vi "HVGEM_AMP_6.2_forDAQ.vi"() -> ()   [LabVIEW 2021]
uses:
  <vilib>/Utility/error.llb/DialogType.ctl
  lib/HVG211.llb/GlobalData.vi
  lib/HVG211.llb/variables.vi
panel:
  in  "path":path=path "Z:/"
  out "refnum":refnum<file>
  out "file open":bool=TRUE caption="Fast"
  in  "ON OLD":bool=TRUE
  out "HV_flag":bool=TRUE
  in  "stop":bool=TRUE caption="Fast"
  out "Currents 2":dbl[](array[numeric]) caption="CURRENTS"
  out "Currents":dbl[](array[numeric]) format="%.2f"
  in  "Trip Control":bool=TRUE caption="SetPreOperational"
  out "OVC":u32[](array[numeric])
  in  "CurrThres":dbl=20.0 caption="uA" min=0.1 max=100.0
  in  "OvflThres":u16=25 caption="number of discharges"
  out "TripCtrl_msg":string="OVCs on 50 samples in 1000 ms:\nTrip if   25 times over   20 uA" caption="INFO_msg"
  in  "dt":u16=20 caption="Time step [ms]" max=5000
  in  "DT":u16=1000 caption="Time window [ms]"
  in  "SpsAcc":bool=TRUE caption="Fast"
  out "Trip Status":u16(ring)=2 items=["DISABLED", "INITIALIZING", "RUNNING", "TRIP"]
  out "slope read":i16=15 caption="Channel" max=2500
  in  "setting 2":i32(ring)=1 items=["TPG", "Planare"]
  out "Currents old":dbl[](array[numeric]) caption="Currents"
  out "Voltages old":dbl[](array[numeric])=[28.0, 28.0, 32.0, 30.0, 29.0, 29.0, 58.0, 0.0, 0.0] caption="Voltages"
  out "sumnew":u16=234
  out "sumold":u16=234
  out "DACOLD":u16[](array[numeric])=[28, 28, 32, 30, 29, 29, 58]
  in  "AVG":u32=100
  out "avg":i16=100 caption="Channel" max=2500
  in  "Slope":u32=15 max=2500
  in  "HV enable switch old":bool=TRUE caption="HV enabled"
  in  "ON":bool
  out "Currents micro":cluster{dbl, dbl, dbl, dbl, dbl, dbl, dbl}(graph)
  out "Wiper":i16[](array[numeric])=[512, 512, 512, 512, 512, 512, 513]
  out "Current_AGC_led":bool
  out "Tramp [s]":u16=5 caption="Channel" max=2500
  out "Tstep [ms]":u16=10 caption="Channel" max=2500
  out "Power Supply Levels":dbl[](array[numeric])=[29.45, 5.357, 3.476, 16.071, 0.384] format="%.1f"
  out "HV enable switch":bool=TRUE caption="HV enabled"
  out "Safety switch":bool=TRUE caption="Cable IN"
  out "FSM_status":u16(ring) items=["IDLE", "RAMPING", "INIT", "ABORTING", "CLEARING", "5", "6", "7", ""]
  out "I_gain_x10":bool[](array[boolean])
  out "HV_on":bool[](array[boolean])=[TRUE, TRUE, TRUE, TRUE, TRUE, TRUE, TRUE, FALSE] caption="HV_ON"
  out "Voltages":dbl[](array[numeric])=[28.0, 28.0, 33.0, 30.0, 29.0, 30.0, 58.0, 0.0, 0.0] caption="VOLTAGES"
  out "TPD_read":bool=TRUE
  out "I_data":cluster{dbl[], dbl[]}[](array[cluster])
  out "V_data":cluster{dbl[], dbl[]}[](array[cluster])
  in  "Ind Gap":dbl=1.0
  in  "Gap 2":dbl=2.0
  in  "Gap 1":dbl=2.0
  in  "Drift Gap":dbl=9.0
  out "STATUS":bool=TRUE
  in  "ID":u8=71
  in  "Limit":u32=2400 min=600 max=3500 step=50
  in  "setting":i32(ring)=4 items=["zero", "test", "field", "600", "900", "1050", "1080", "1090", "1100", "1110", "1120", "1130", "1140", "1160", "1200", "1240", "1260", "1280", "1300", "1320"]
  in  "Apply":bool
  out "time":u32=185445358 format="%#.0f"
  in  "Write data":bool
  out "Run":i32=5
  out "Gain":u32=88
  out "String":string="FILLING  HISTOS"
  out "Vd":dbl=58.0
  out "Vt1":dbl=29.0
  out "Vt2":dbl=33.0
  out "Vi":dbl=28.0
  out "G3":dbl=28.0
  out "G1":dbl=30.0
  out "G2":dbl=30.0
  out "Ed":dbl=0.06444444444444444 format="%.1f"
  out "Ei":dbl=0.28 format="%.1f"
  out "Et2":dbl=0.165 format="%.1f"
  out "Et1":dbl=0.145 format="%.1f"
  out "Fields kV/cm":cluster{dbl, dbl, dbl, dbl}(graph)={0.06444444444444444, 0.145, 0.165, 0.28}
  out "GEM Volt":cluster{dbl, dbl, dbl}(graph)={30.0, 30.0, 28.0}
  out "DACNEW":u16[](array[numeric])=[28, 28, 32, 30, 29, 29, 58]
  out "ERROR":errorcluster={"status"=TRUE, "code"=-10, "source"="Handle is invalid"}
  out "PreOperational":bool
  out "Operational":bool=TRUE
  out "OPERATION ERROR":errorcluster
  out "gi":dbl=100.0 format="%.2f"
  out "gt2":dbl=200.0 format="%.2f"
  out "gt1":dbl=200.0 format="%.2f"
  out "gd":dbl=900.0 format="%.2f"
  in  "Ind":dbl=0.28 caption="Induction Field (kV/cm)" min=0.0 max=10.0 step=0.1 format="%.1f"
  in  "T2":dbl=0.16 caption="Transfer Field 2 (kV/cm)" min=0.0 max=4.0 step=0.1 format="%.1f"
  in  "T1":dbl=0.145 caption="Transfer Field 1(kV/cm)" min=0.0 max=4.0 step=0.1 format="%.1f"
  in  "Drift":dbl=0.06444444444444444 caption="Drift Field (kV/cm)" min=0.0 max=4.0 step=0.1 format="%.2f"
  in  "VG3":i16=28 caption="Vg3 (Volt)" min=0 max=600 step=5
  in  "VG2":i16=30 caption="Vg2 (Volt)" min=0 max=600 step=5
  in  "VG1":i16=29 caption="Vg1 (Volt)" min=0 max=600 step=5
  out "t0":u32=1496531
  # "HV GEM AMP 6.2"
  # "HV ON"
  # "Volt"
  # "kV/cm"
  # "kV/cm"
  # "Volt"
  # "GAP(mm)"
  # "EI         G3       ET2      G2      ET1      G1       ED"
  # "TEMP"
  # "PS1"
  # "PS2"
  # "PS3"
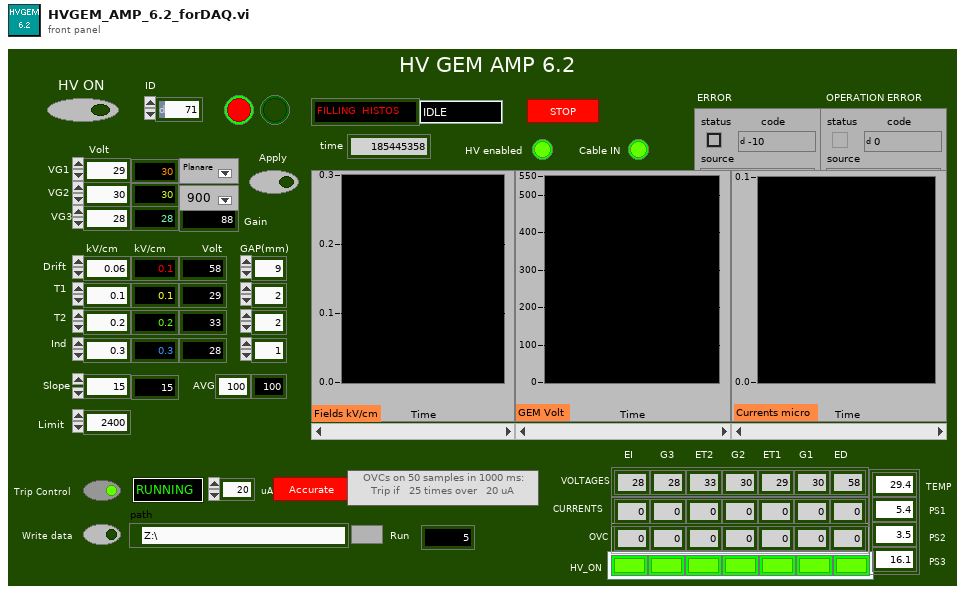
[diagram p1: front panel]
types:
  T1 = enum16{"open", "open or create", "create or replace", "create", "open (read only)"}
  T2 = typedef "DialogType.ctl" = u16
  T3 = cluster{"Safety switch":bool, "HV disable switch":bool, "HV_on":bool[], "I_gain_x10":bool[], "FSM_status":u16, "0x2020":dbl[], "Tstep":u16, "Tramp":u16, "Average":i16, "Current AGC":bool, "Wiper":i16[], "Slope [V/s]":i16}
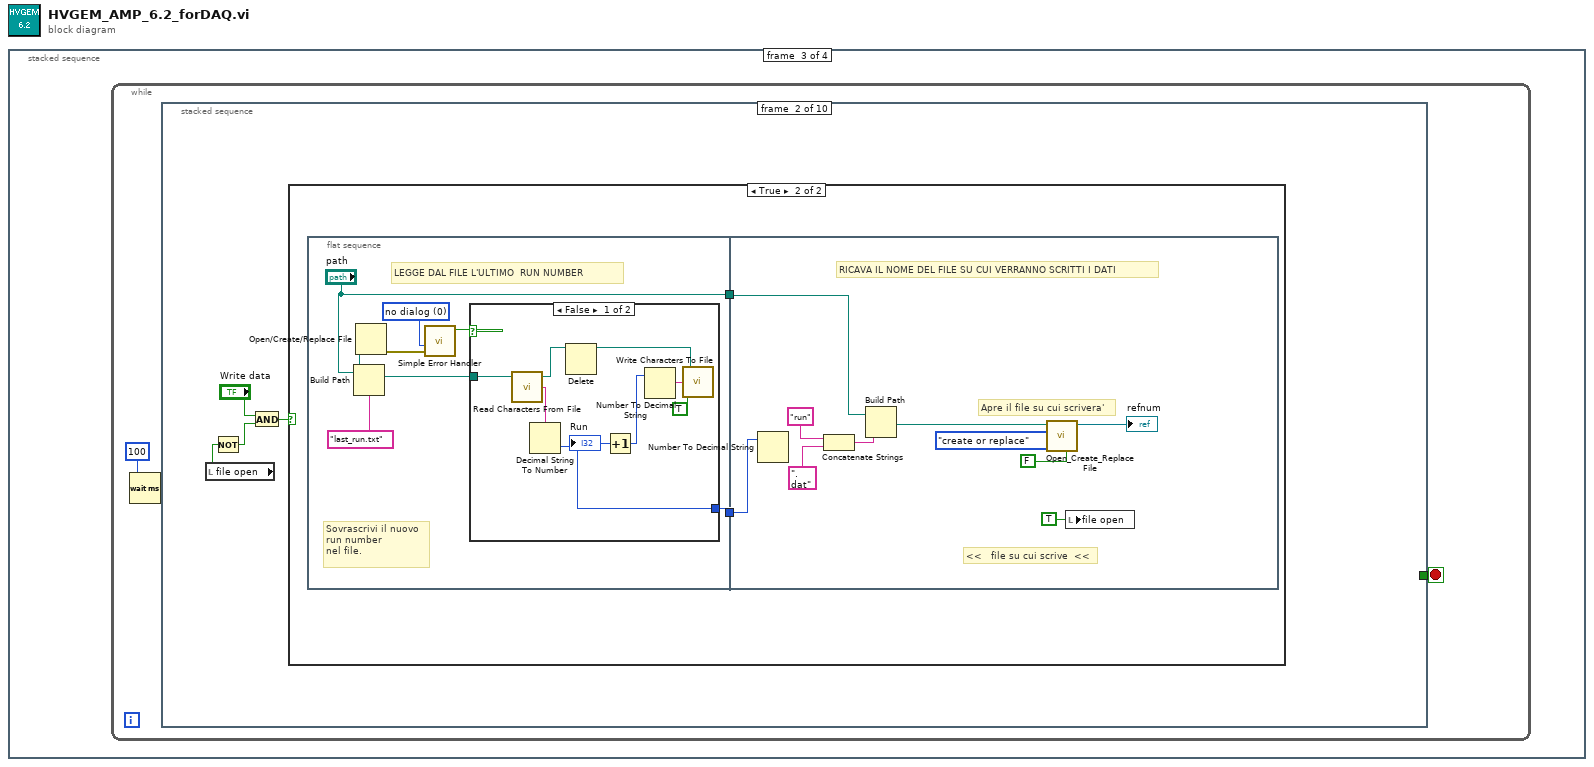
[diagram p0: block diagram]
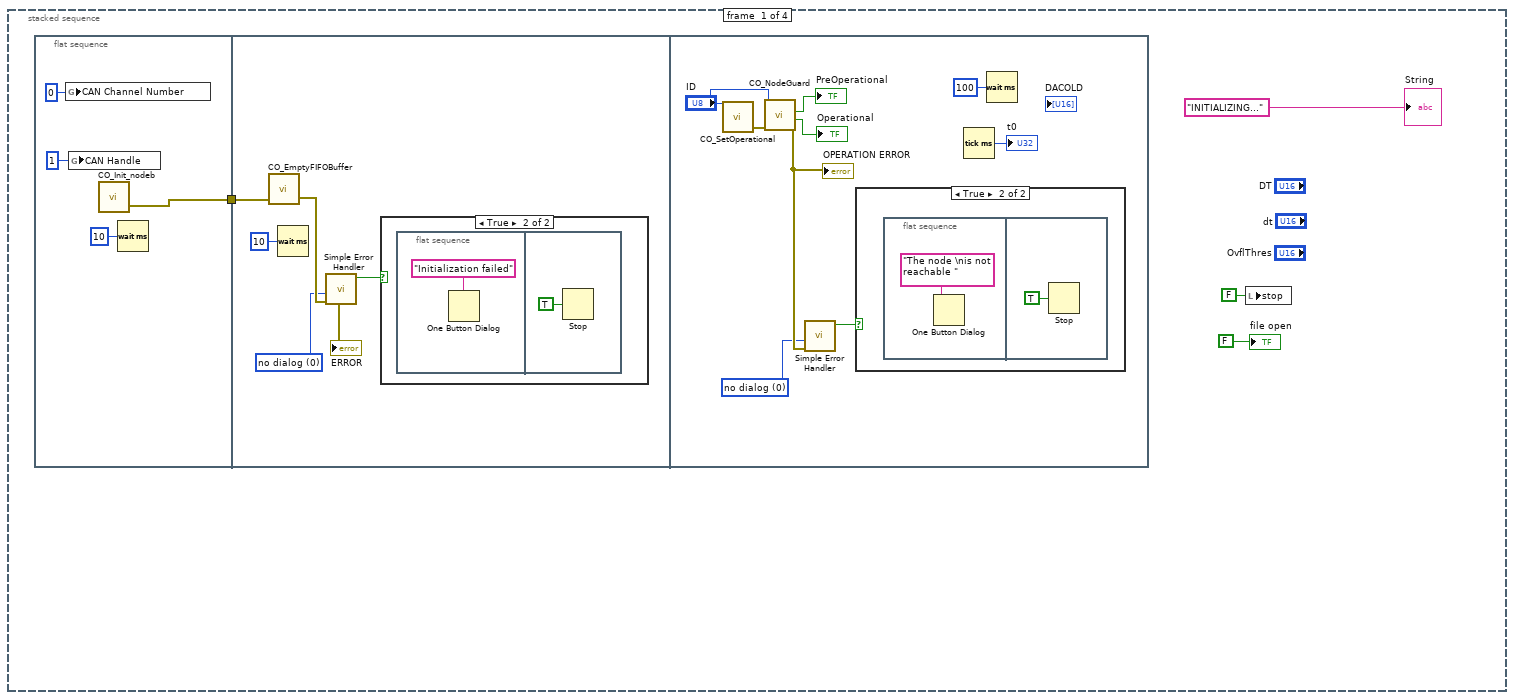
[diagram p2: hidden frame]
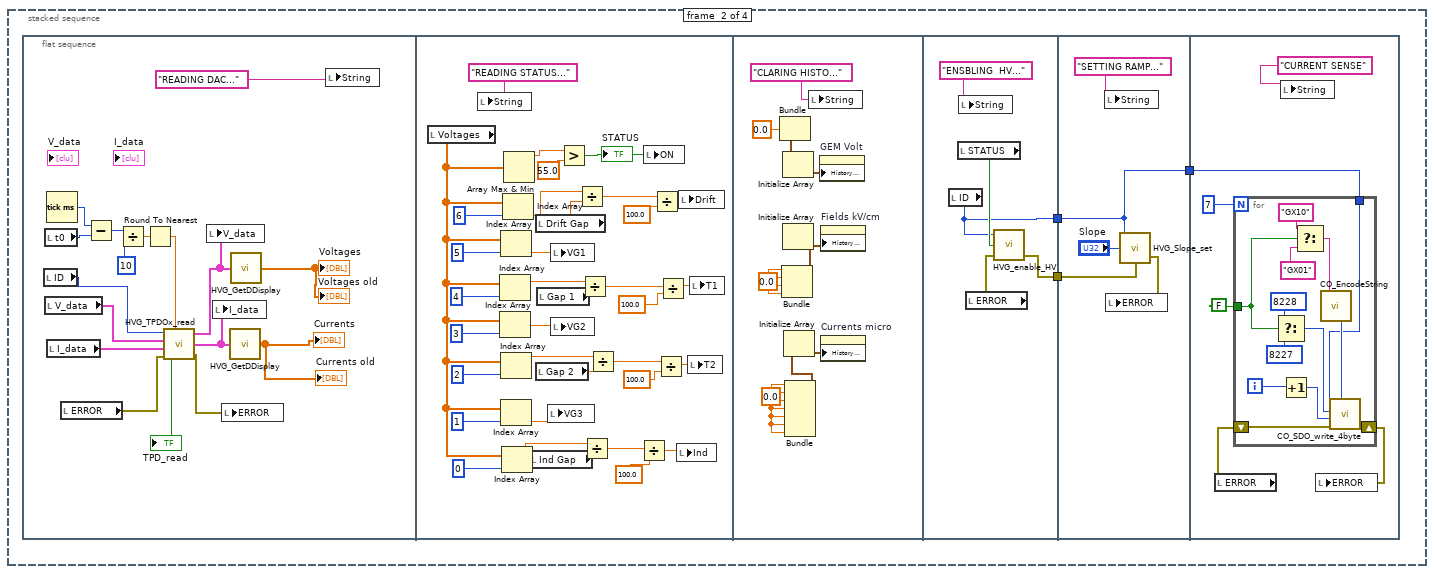
[diagram p5: hidden frame]
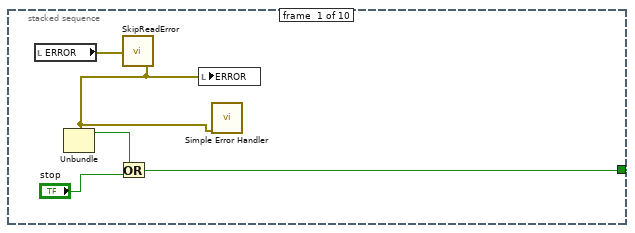
[diagram p6: hidden frame]
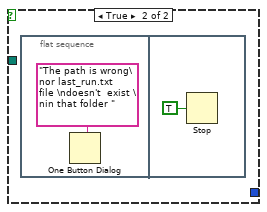
[diagram p8: hidden frame]
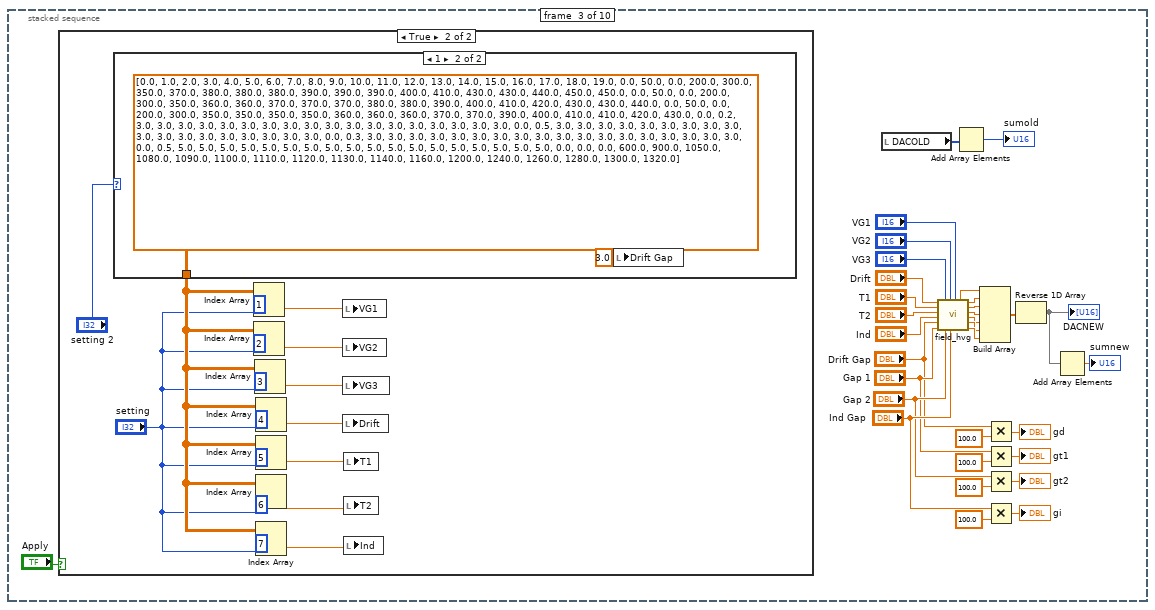
[diagram p9: hidden frame]
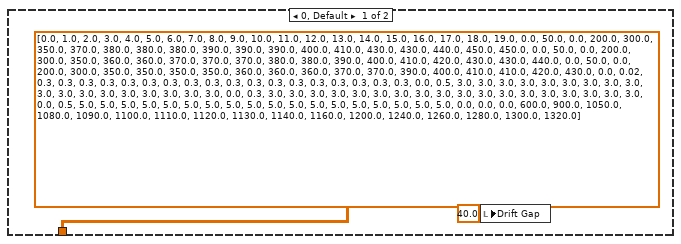
[diagram p11: hidden frame]
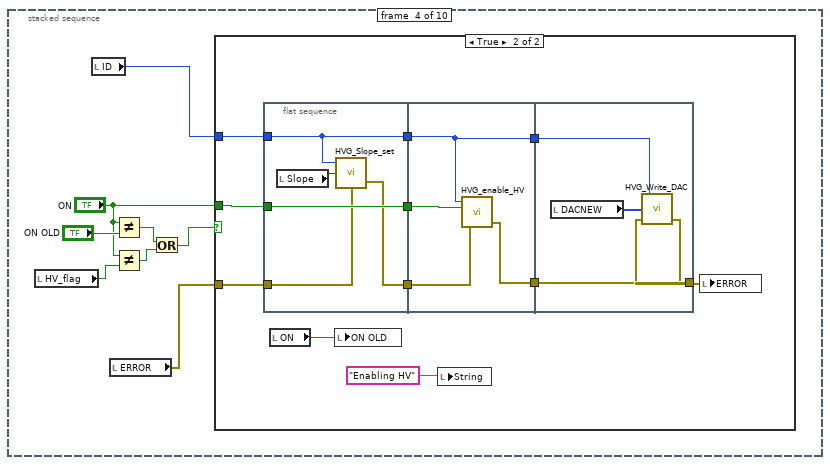
[diagram p12: hidden frame]
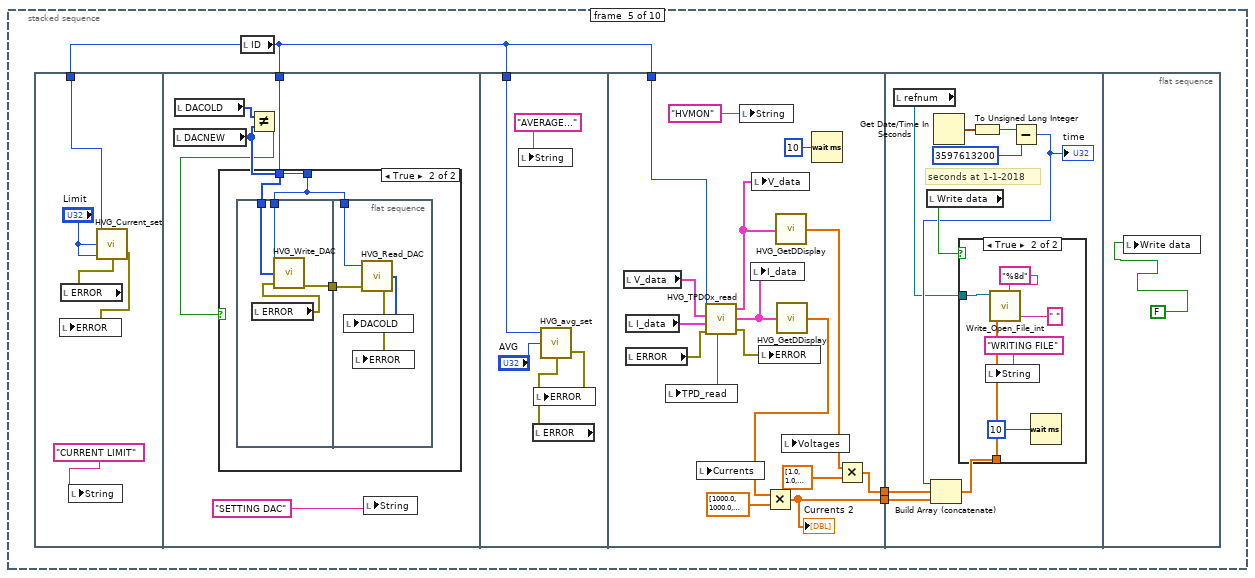
[diagram p14: hidden frame]
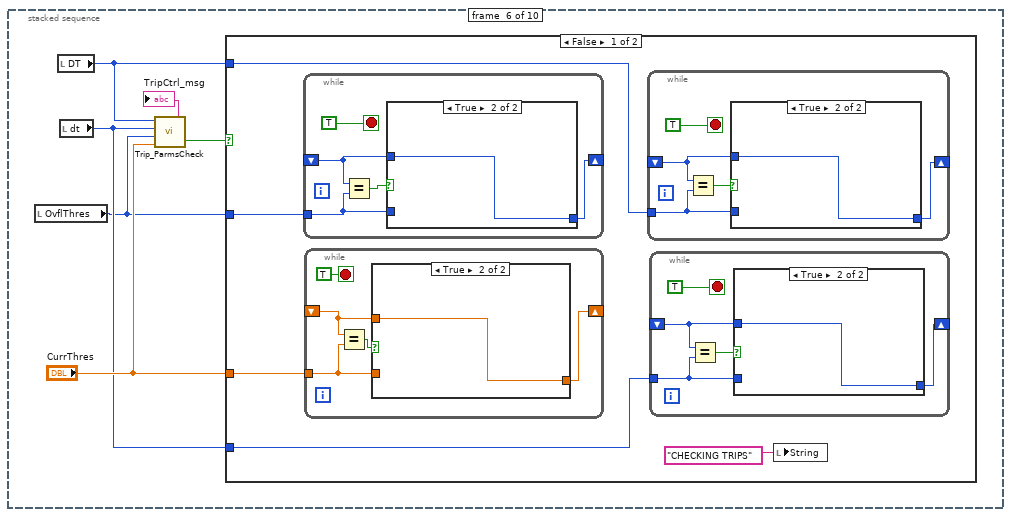
[diagram p17: hidden frame]
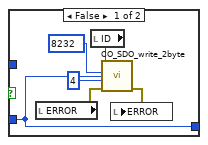
[diagram p18: hidden frame]
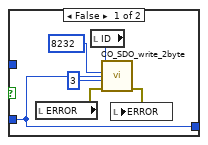
[diagram p19: hidden frame]
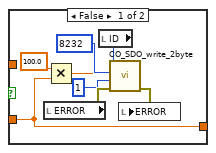
[diagram p20: hidden frame]
diagram:
  n1 = stacked-sequence {
    frame #0 {
      (unwired) FALSE ("Boolean 2")
      n2 = flat-sequence {
        tunnel: [w7] -> w3
        tunnel: w3 -> [w12]
        frame #0 {
          n3 = global write "GlobalData.vi" "CAN Channel Number"(0 ("CAN Handle")) -> ()
          n4 = global write "GlobalData.vi" "CAN Handle"(1 ("CAN Handle")) -> ()
          n5 = call "CO_Init_nodeb.vi"() -> ("error out"=w7:errorcluster)  [unwired: 3 in]
          n6 = Wait (ms)(milliseconds to wait=u32 10) -> ()  [unwired: 1 out]
        }
        frame #1 {
          w9 = T2 0 items=["no dialog", "OK message", "continue or stop message", "OK message + warnings", "continue/stop + warnings"] ("type of dialog (OK msg:1)")
          n7 = call "CO_EmptyFIFOBuffer.vi"("error in"=w12) -> ("error out"=w10:errorcluster)  [unwired: 2 in]
          "ERROR" <- w10
          n8 = Wait (ms)(milliseconds to wait=u32 10) -> ()  [unwired: 1 out]
          n9 = call <vilib>:"Simple Error Handler.vi"("type of dialog (OK msg:1)"=w9, "error in (no error)"=w10) -> ("error?"=w11:bool)  [unwired: 3 in, 4 out]
          n10 = case shown="True" w11 {
            frame False {
            }
            frame True {
              n11 = flat-sequence {
                frame #0 {
                  n12 = One Button Dialog(message="Initialization failed") -> ()  [unwired: 1 in, 1 out]
                }
                frame #1 {
                  n13 = Stop(stop? (T)=TRUE) -> ()
                }
              }
            }
          }
        }
        frame #2 {
          w16 = T2 0 items=["no dialog", "OK message", "continue or stop message", "OK message + warnings", "continue/stop + warnings"] ("type of dialog (OK msg:1)")
          n14 = call "CO_SetOperational.vi"("ID"="ID") -> ("error out"=w21:errorcluster)  [unwired: 4 in]
          n15 = call "CO_NodeGuard.vi"("error in (no error)"=w21, "ID"="ID") -> ("error out"=w18:errorcluster, "Operational"=→"Operational":bool, "PreOperational"=→"PreOperational":bool)  [unwired: 3 in, 2 out]
          "OPERATION ERROR" <- w18
          n16 = call <vilib>:"Simple Error Handler.vi"("type of dialog (OK msg:1)"=w16, "error in (no error)"=w18) -> ("error?"=w17:bool)  [unwired: 3 in, 4 out]
          n17 = case shown="True" w17 {
            frame False {
            }
            frame True {
              n18 = flat-sequence {
                frame #0 {
                  n19 = One Button Dialog(message="The node \nis not reachable ") -> ()  [unwired: 1 in, 1 out]
                }
                frame #1 {
                  n20 = Stop(stop? (T)=TRUE) -> ()
                }
              }
            }
          }
          n21 = Tick Count (ms)() -> (millisecond timer value=→"t0":u32)
          n22 = Wait (ms)(milliseconds to wait=u32 100) -> ()  [unwired: 1 out]
        }
      }
      n23 = local write "stop"(FALSE ("stop")) -> ()
      "String" <- "INITIALIZING..." ("String")
      "file open" <- FALSE
    }
    frame #1 {
      n24 = flat-sequence {
        tunnel: [w93] -> w28
        tunnel: [w92] -> w27
        tunnel: [w98] -> w29
        tunnel: w28 -> [w98]
        tunnel: w27 -> [w97]
        tunnel: w29 -> [w102]
        frame #0 {
          n25 = local read "ID"() -> (w32:u8)
          n26 = local read "t0"() -> (w39:u32)
          n27 = local read "V_data"() -> (w45:cluster{dbl[], dbl[]}[])
          n28 = Tick Count (ms)() -> (millisecond timer value=w40:u32)
          n29 = local read "I_data"() -> (w44:cluster{dbl[], dbl[]}[])
          n30 = local read "ERROR"() -> (w42:errorcluster)
          n31 = Subtract(x=w40, y=w39) -> (x-y=w38:u32)
          n32 = Divide(x=w38, y=u32 10) -> (x/y=w36:dbl)
          n33 = Round To Nearest(number=w36) -> (nearest integer value=w35:dbl)
          n34 = call "HVG_TPDOx_read.vi"("ID"=w32, "T"=w35, "V_data_in"=w45, "I_data_in"=w44, "Error in"=w42) -> ("Data_read"=→"TPD_read":bool, "V_data_out"=w33:cluster{dbl[], dbl[]}[], "I_data_out"=w34:cluster{dbl[], dbl[]}[], "Error out"=w43:errorcluster)
          n35 = local write "V_data"(w33) -> ()
          n36 = local write "I_data"(w34) -> ()
          n37 = local write "ERROR"(w43) -> ()
          n38 = call "HVG_GetDDisplay.vi"("I_data_out"=w34) -> ("Array"=→"Currents old" →"Currents":dbl[])
          n39 = call "HVG_GetDDisplay.vi"("I_data_out"=w33) -> ("Array"=→"Voltages" →"Voltages old":dbl[])
          n40 = local write "String"("READING DAC..." ("String")) -> ()
        }
        frame #1 {
          n41 = local read "Voltages"() -> (w73:dbl[])
          n42 = local write "String"("READING STATUS..." ("String")) -> ()
          n43 = Index Array(array=w73, index=4) -> (element=w64:dbl)
          n44 = Index Array(array=w73, index=3) -> (element=w71:dbl)
          n45 = Index Array(array=w73, index=5) -> (element=w72:dbl)
          n46 = Index Array(array=w73, index=2) -> (element=w63:dbl)
          n47 = Index Array(array=w73, index=1) -> (element=w70:dbl)
          n48 = Index Array(array=w73, index=0) -> (element=w62:dbl)
          n49 = Index Array(array=w73, index=6) -> (element=w69:dbl)
          n50 = Array Max & Min(array=w73) -> (max value=w48:dbl)  [unwired: 3 out]
          n51 = local read "Ind Gap"() -> (w59:dbl)
          n52 = local read "Drift Gap"() -> (w68:dbl)
          n53 = local read "Gap 2"() -> (w60:dbl)
          n54 = local read "Gap 1"() -> (w61:dbl)
          n55 = local write "VG3"(w70) -> ()
          n56 = local write "VG1"(w72) -> ()
          n57 = local write "VG2"(w71) -> ()
          n58 = Greater?(x=w48, y=55.0) -> (0:w49:bool)
          "STATUS" <- w49
          n59 = Divide(x=w69, y=w68) -> (x/y=w66:dbl)
          n60 = Divide(x=w64, y=w61) -> (x/y=w58:dbl)
          n61 = Divide(x=w62, y=w59) -> (x/y=w54:dbl)
          n62 = Divide(x=w63, y=w60) -> (x/y=w55:dbl)
          n63 = Divide(x=w54, y=100.0) -> (x/y=w52:dbl)
          n64 = local write "ON"(w49) -> ()
          n65 = Divide(x=w66, y=100.0) -> (x/y=w65:dbl)
          n66 = Divide(x=w55, y=100.0) -> (x/y=w51:dbl)
          n67 = Divide(x=w58, y=100.0) -> (x/y=w50:dbl)
          n68 = local write "Ind"(w52) -> ()
          n69 = local write "Drift"(w65) -> ()
          n70 = local write "T2"(w51) -> ()
          n71 = local write "T1"(w50) -> ()
        }
        frame #2 {
          w84 = 0.0
          w86 = 0.0
          w89 = 0.0
          n72 = Bundle(w86, w86, w86) -> (w88:cluster{dbl, dbl, dbl})  [unwired: 1 in]
          n73 = Bundle(w89, w89, w89, w89) -> (w91:cluster{dbl, dbl, dbl, dbl})  [unwired: 1 in]
          n74 = Initialize Array(w88) -> (w87:cluster{dbl, dbl, dbl}[])  [unwired: 1 in]
          n75 = Initialize Array(w91) -> (w90:cluster{dbl, dbl, dbl, dbl}[])  [unwired: 1 in]
          n76 = Bundle(w84, w84, w84, w84, w84, w84, w84) -> (w83:cluster{dbl, dbl, dbl, dbl, dbl, dbl, dbl})  [unwired: 1 in]
          n77 = Initialize Array(w83) -> (w82:cluster{dbl, dbl, dbl, dbl, dbl, dbl, dbl}[])  [unwired: 1 in]
          n78 = local write "String"("CLARING HISTO..." ("String")) -> ()
          n79 = property on="GEM Volt" class="WFChart (strict)"("History Data"=w87) -> ()  [unwired: 2 in, 2 out]
          n80 = property on="Fields kV/cm" class="WFChart (strict)"("History Data"=w90) -> ()  [unwired: 2 in, 2 out]
          n81 = property on="Currents micro" class="WFChart (strict)"("History Data"=w82) -> ()  [unwired: 2 in, 2 out]
        }
        frame #3 {
          n82 = local read "ID"() -> (w93:u8)
          n83 = local read "STATUS"() -> (w94:bool)
          n84 = local write "String"("ENSBLING  HV..." ("String")) -> ()
          n85 = local read "ERROR"() -> (w95:errorcluster)
          n86 = call "HVG_enable_HV.vi"("Error_In"=w95, "Enable_all"=w94, "ID"=w93) -> ("Error_Out"=w92:errorcluster)  [unwired: 2 in]
        }
        frame #4 {
          n87 = local write "String"("SETTING RAMP..." ("String")) -> ()
          n88 = call "HVG_Slope_set.vi"("Error_In"=w97, "slope"="Slope", "ID"=w98) -> ("Error_Out"=w99:errorcluster)  [unwired: 2 in]
          n89 = local write "ERROR"(w99) -> ()
        }
        frame #5 {
          n90 = local read "ERROR"() -> (w104:errorcluster)
          n91 = for {
            N: 7 -> [_]
            shift-right: [w120] -> w103
            shift-left: w104 -> [w119]
            tunnel: FALSE ("Current_AGC") -> [w109]
            tunnel: w102 -> [w108]
            i -> [w115]
            n92 = Select(t=8228, s=w109, f=8227 ("t")) -> (s? t:f=w116:i32)
            n93 = Increment(x=w115) -> (x+1=w114:i32)
            n94 = Select(t="GX10", s=w109, f="GX01" ("t")) -> (s? t:f=w110:string)
            n95 = call "CO_EncodeString.vi"("String"=w110) -> ("Value"=w111:u32)  [unwired: 1 out]
            n96 = call "CO_SDO_write_4byte.vi"("Value"=w111, "error in (no error)"=w119, "SubIndex"=w114, "Index"=w116, "ID"=w108) -> ("error out"=w120:errorcluster)  [unwired: 3 in, 1 out]
          }
          n97 = local write "String"("CURRENT SENSE" ("String")) -> ()
          n98 = local write "ERROR"(w103) -> ()
        }
      }
    }
    frame #2 {
      n99 = while {
        stop <- w122 stop-if-true
        n100 = Wait (ms)(milliseconds to wait=u32 100) -> ()  [unwired: 1 out]
        n101 = stacked-sequence {
          tunnel: [w125 _ _ _ _ _ _ _ _ _] -> w122
          frame #0 {
            n102 = local read "ERROR"() -> (w127:errorcluster)
            n103 = call "SkipReadError.vi"("error in"=w127) -> ("error out"=w124:errorcluster)
            n104 = Unbundle(w124) -> ("status"=w126:bool)  [unwired: 2 out]
            n105 = Or(x=w126, y="stop") -> (x .or. y?=w125:bool)
            n106 = local write "ERROR"(w124) -> ()
            n107 = call <vilib>:"Simple Error Handler.vi"("error in (no error)"=w124) -> ()  [unwired: 4 in, 5 out]
          }
          frame #1 {
            n108 = local read "file open"() -> (w130:bool)
            n109 = Not(x=w130) -> (.not. x?=w129:bool)
            n110 = And(x="Write data", y=w129) -> (x .and. y?=w128:bool)
            n111 = case shown="True" w128 {
              frame False {
              }
              frame True {
                n112 = flat-sequence {
                  tunnel: [w140] -> w133
                  tunnel: ["path"] -> w132
                  tunnel: w133 -> [w157]
                  tunnel: w132 -> [w152]
                  frame #0 {
                    w134 = T2 0 items=["no dialog", "OK message", "continue or stop message", "OK message + warnings", "continue/stop + warnings"] ("type of dialog (OK msg:1)")
                    # "Sovrascrivi il nuovo\nrun number\nnel file."
                    # "LEGGE DAL FILE L'ULTIMO  RUN NUMBER"
                    n113 = Build Path(base path="path", name or relative path="last_run.txt") -> (appended path=w137:path)
                    n114 = Open/Create/Replace File(file path (use dialog)=w137) -> (error out=w136:errorcluster)  [unwired: 5 in, 2 out]
                    n115 = call <vilib>:"Simple Error Handler.vi"("type of dialog (OK msg:1)"=w134, "error in (no error)"=w136) -> ("error?"=w135:bool)  [unwired: 3 in, 4 out]
                    n116 = case shown="False" w135 {
                      tunnel: [w143 _] -> w140
                      tunnel: w137 -> [w141 _]
                      frame False {
                        n117 = call <vilib>:"Read Characters From File.vi"("file path (dialog if empty)"=w141) -> ("new file path (NotAPath if cancelled)"=w142:path, "character string"=w144:string)  [unwired: 5 in, 2 out]
                        n118 = Decimal String To Number(string=w144) -> (number=w143:i32)  [unwired: 2 in, 1 out]
                        "Run" <- w143
                        n119 = Delete(path (use dialog)=w142) -> (deleted path=w148:path)  [unwired: 4 in, 2 out]
                        n120 = Increment(x=w143) -> (x+1=w147:i32)
                        n121 = Number To Decimal String(number=w147) -> (decimal integer string=w145:string)  [unwired: 1 in]
                        n122 = call <vilib>:"Write Characters To File.vi"("append to file? (new file:F)"=TRUE, "character string"=w145, "file path (dialog if empty)"=w148) -> ()  [unwired: 2 in, 1 out]
                      }
                      frame True {
                        n123 = flat-sequence {
                          frame #0 {
                            n124 = One Button Dialog(message="The path is wrong\nor last_run.txt file \ndoesn't  exist \nin that folder ") -> ()  [unwired: 1 in, 1 out]
                          }
                          frame #1 {
                            n125 = Stop(stop? (T)=TRUE) -> ()
                          }
                        }
                      }
                    }
                  }
                  frame #1 {
                    # "Apre il file su cui scrivera'"
                    # "<<   file su cui scrive  <<"
                    # "RICAVA IL NOME DEL FILE SU CUI VERRANNO SCRITTI I DATI"
                    n126 = Number To Decimal String(number=w157) -> ()  [unwired: 1 in, 1 out]
                    n127 = Concatenate Strings("run" ("string"), ".dat" ("string")) -> (w160:string)
                    n128 = Build Path(base path=w152, name or relative path=w160) -> (appended path=w158:path)
                    n129 = call <vilib>:"Open_Create_Replace File.vi"("advisory dialog? (display:T)"=FALSE, "function (open:0)"=T1."create or replace", "file path"=w158) -> ("refnum"=→"refnum":refnum<file>)  [unwired: 5 in, 3 out]
                    n130 = local write "file open"(TRUE ("file open")) -> ()
                  }
                }
              }
            }
          }
          frame #2 {
            n131 = case shown="True" "Apply" {
              frame False {
              }
              frame True {
                n132 = case shown="1" "setting 2" {
                  tunnel: [dbl[][] [[0.0, 1.0, 2.0, 3.0, 4.0, 5.0, 6.0, 7.0, 8.0, 9.0, 10.0, 11.0, 12.0, 13.0, 14.0, 15.0, 16.0, 17.0, 18.0, 19.0], [0.0, 50.0, 0.0, 200.0, 300.0, 350.0, 370.0, 380.0, 380.0, 380.0, 390.0, 390.0, 390.0, 400.0, 410.0, 430.0, 430.0, 440.0, 450.0, 450.0], [0.0, 50.0, 0.0, 200.0, 300.0, 350.0, 360.0, 360.0, 370.0, 370.0, 370.0, 380.0, 380.0, 390.0, 400.0, 410.0, 420.0, 430.0, 430.0, 440.0], [0.0, 50.0, 0.0, 200.0, 300.0, 350.0, 350.0, 350.0, 350.0, 360.0, 360.0, 360.0, 370.0, 370.0, 390.0, 400.0, 410.0, 410.0, 420.0, 430.0], [0.0, 0.02, 0.3, 0.3, 0.3, 0.3, 0.3, 0.3, 0.3, 0.3, 0.3, 0.3, 0.3, 0.3, 0.3, 0.3, 0.3, 0.3, 0.3, 0.3], [0.0, 0.5, 3.0, 3.0, 3.0, 3.0, 3.0, 3.0, 3.0, 3.0, 3.0, 3.0, 3.0, 3.0, 3.0, 3.0, 3.0, 3.0, 3.0, 3.0], [0.0, 0.3, 3.0, 3.0, 3.0, 3.0, 3.0, 3.0, 3.0, 3.0, 3.0, 3.0, 3.0, 3.0, 3.0, 3.0, 3.0, 3.0, 3.0, 3.0], [0.0, 0.5, 5.0, 5.0, 5.0, 5.0, 5.0, 5.0, 5.0, 5.0, 5.0, 5.0, 5.0, 5.0, 5.0, 5.0, 5.0, 5.0, 5.0, 5.0], [0.0, 0.0, 0.0, 600.0, 900.0, 1050.0, 1080.0, 1090.0, 1100.0, 1110.0, 1120.0, 1130.0, 1140.0, 1160.0, 1200.0, 1240.0, 1260.0, 1280.0, 1300.0, 1320.0]] dbl[][] [[0.0, 1.0, 2.0, 3.0, 4.0, 5.0, 6.0, 7.0, 8.0, 9.0, 10.0, 11.0, 12.0, 13.0, 14.0, 15.0, 16.0, 17.0, 18.0, 19.0], [0.0, 50.0, 0.0, 200.0, 300.0, 350.0, 370.0, 380.0, 380.0, 380.0, 390.0, 390.0, 390.0, 400.0, 410.0, 430.0, 430.0, 440.0, 450.0, 450.0], [0.0, 50.0, 0.0, 200.0, 300.0, 350.0, 360.0, 360.0, 370.0, 370.0, 370.0, 380.0, 380.0, 390.0, 400.0, 410.0, 420.0, 430.0, 430.0, 440.0], [0.0, 50.0, 0.0, 200.0, 300.0, 350.0, 350.0, 350.0, 350.0, 360.0, 360.0, 360.0, 370.0, 370.0, 390.0, 400.0, 410.0, 410.0, 420.0, 430.0], [0.0, 0.2, 3.0, 3.0, 3.0, 3.0, 3.0, 3.0, 3.0, 3.0, 3.0, 3.0, 3.0, 3.0, 3.0, 3.0, 3.0, 3.0, 3.0, 3.0], [0.0, 0.5, 3.0, 3.0, 3.0, 3.0, 3.0, 3.0, 3.0, 3.0, 3.0, 3.0, 3.0, 3.0, 3.0, 3.0, 3.0, 3.0, 3.0, 3.0], [0.0, 0.3, 3.0, 3.0, 3.0, 3.0, 3.0, 3.0, 3.0, 3.0, 3.0, 3.0, 3.0, 3.0, 3.0, 3.0, 3.0, 3.0, 3.0, 3.0], [0.0, 0.5, 5.0, 5.0, 5.0, 5.0, 5.0, 5.0, 5.0, 5.0, 5.0, 5.0, 5.0, 5.0, 5.0, 5.0, 5.0, 5.0, 5.0, 5.0], [0.0, 0.0, 0.0, 600.0, 900.0, 1050.0, 1080.0, 1090.0, 1100.0, 1110.0, 1120.0, 1130.0, 1140.0, 1160.0, 1200.0, 1240.0, 1260.0, 1280.0, 1300.0, 1320.0]]] -> w195
                  frame 0, Default {
                    n133 = local write "Drift Gap"(40.0 ("Drift Gap")) -> ()
                  }
                  frame 1 {
                    n134 = local write "Drift Gap"(3.0 ("Drift Gap")) -> ()
                  }
                }
                n135 = Index Array(array=w195, index (row)=1 ("index"), index (col)="setting") -> (element=w208:dbl)
                n136 = Index Array(array=w195, index (row)=2 ("index"), index (col)="setting") -> (element=w201:dbl)
                n137 = Index Array(array=w195, index (row)=3 ("index"), index (col)="setting") -> (element=w200:dbl)
                n138 = Index Array(array=w195, index (row)=4 ("index"), index (col)="setting") -> (element=w199:dbl)
                n139 = Index Array(array=w195, index (row)=5 ("index"), index (col)="setting") -> (element=w198:dbl)
                n140 = Index Array(array=w195, index (row)=6 ("index"), index (col)="setting") -> (element=w197:dbl)
                n141 = Index Array(array=w195, index (row)=7 ("index"), index (col)="setting") -> (element=w196:dbl)
                n142 = local write "VG1"(w208) -> ()
                n143 = local write "VG2"(w201) -> ()
                n144 = local write "VG3"(w200) -> ()
                n145 = local write "Drift"(w199) -> ()
                n146 = local write "T1"(w198) -> ()
                n147 = local write "T2"(w197) -> ()
                n148 = local write "Ind"(w196) -> ()
              }
            }
            n149 = local read "DACOLD"() -> (w164:u16[])
            n150 = call "field_hvg.vi"("Drift Field (kV/cm)"="Drift", "Transfer Field 1(kV/cm)"="T1", "Transfer Field 2 (kV/cm)"="T2", "Induction Field (kV/cm)"="Ind", "Drift Gap (mm)"="Drift Gap", "Transfer Gap 1 (mm)"="Gap 1", "Vg3 (Volt)"="VG3", "Transfer Gap 2 (mm)"="Gap 2", "Vg2 (Volt)"="VG2", "Induction Gap"="Ind Gap", "Vg1 (Volt)"="VG1") -> ("Cathode"=w174:dbl, "Vg1 up"=w175:dbl, "Vg1 down"=w176:dbl, "Vg2 up"=w177:dbl, "Vg2 down"=w178:dbl, "Vg3 up"=w179:dbl, "Vg3 down"=w180:dbl)  [unwired: 1 in, 1 out]
            n151 = Add Array Elements(numeric array=w164) -> (sum=→"sumold":u16)
            n152 = Build Array(w174, w175, w176, w177, w178, w179, w180) -> (w181:dbl[])
            n153 = Multiply(x="Drift Gap", y=100.0) -> (x*y=→"gd":dbl)
            n154 = Multiply(x="Gap 1", y=100.0) -> (x*y=→"gt1":dbl)
            n155 = Multiply(x="Gap 2", y=100.0) -> (x*y=→"gt2":dbl)
            n156 = Multiply(x="Ind Gap", y=100.0) -> (x*y=→"gi":dbl)
            n157 = Reverse 1D Array(array=w181) -> (reversed array=w161:dbl[])
            "DACNEW" <- w161
            n158 = Add Array Elements(numeric array=w161) -> (sum=→"sumnew":dbl)
          }
          frame #3 {
            n159 = local read "HV_flag"() -> (w218:bool)
            n160 = local read "ID"() -> (w221:u8)
            n161 = local read "ERROR"() -> (w220:errorcluster)
            n162 = Not Equal?(x="ON", y="ON OLD") -> (x != y?=w215:bool)
            n163 = Not Equal?(x="ON", y=w218) -> (x != y?=w216:bool)
            n164 = Or(x=w215, y=w216) -> (x .or. y?=w214:bool)
            n165 = case shown="True" w214 {
              tunnel: w221 -> [_ w227]
              tunnel: w220 -> [_ w226]
              tunnel: "ON" -> [_ w223]
              frame False {
              }
              frame True {
                n166 = flat-sequence {
                  tunnel: w227 -> [w234]
                  tunnel: w226 -> [w236]
                  tunnel: w223 -> [w237]
                  tunnel: [w237] -> w232
                  tunnel: [w234] -> w231
                  tunnel: [w235] -> w230
                  tunnel: w232 -> [w241]
                  tunnel: w231 -> [w238]
                  tunnel: w230 -> [w240]
                  tunnel: [w239] -> w229
                  tunnel: [w238] -> w228
                  tunnel: [w242] -> w224
                  tunnel: w229 -> [w243]
                  tunnel: w228 -> [w245]
                  frame #0 {
                    n167 = local read "Slope"() -> (w233:u32)
                    n168 = call "HVG_Slope_set.vi"("Error_In"=w236, "slope"=w233, "ID"=w234) -> ("Error_Out"=w235:errorcluster)  [unwired: 2 in]
                  }
                  frame #1 {
                    n169 = call "HVG_enable_HV.vi"("Error_In"=w240, "Enable_all"=w241, "ID"=w238) -> ("Error_Out"=w239:errorcluster)  [unwired: 2 in]
                  }
                  frame #2 {
                    n170 = local read "DACNEW"() -> (w244:u16[])
                    n171 = call "HVG_Write_DAC.vi"("Error_In"=w243, "DACnew"=w244, "ID"=w245) -> ("Error_Out"=w242:errorcluster)  [unwired: 2 in]
                  }
                }
                n172 = local read "ON"() -> (w222:bool)
                n173 = local write "ON OLD"(w222) -> ()
                n174 = local write "String"("Enabling HV" ("String")) -> ()
                n175 = local write "ERROR"(w224) -> ()
              }
            }
          }
          frame #4 {
            n176 = flat-sequence {
              tunnel: w246 -> [w252]
              tunnel: w246 -> [w258]
              tunnel: w246 -> [w272]
              tunnel: w246 -> [w282]
              tunnel: [w277] -> w248
              tunnel: [w275] -> w247
              tunnel: w248 -> [w294]
              tunnel: w247 -> [w293]
              frame #0 {
                n177 = local read "ERROR"() -> (w250:errorcluster)
                n178 = local write "String"("CURRENT LIMIT" ("String")) -> ()
                n179 = call "HVG_Current_set.vi"("Error_In"=w250, "limit_7 [mV]"="Limit", "limit_1-6"="Limit", "ID"=w252) -> ("Error_Out"=w249:errorcluster)  [unwired: 1 in]
                n180 = local write "ERROR"(w249) -> ()
              }
              frame #1 {
                n181 = local read "DACNEW"() -> (w256:u16[])
                n182 = local read "DACOLD"() -> (w257:u16[])
                n183 = Not Equal?(x=w257, y=w256) -> (x != y?=w255:bool)
                n184 = case shown="True" w255 {
                  tunnel: w258 -> [_ w259]
                  tunnel: w256 -> [_ w261]
                  frame False {
                  }
                  frame True {
                    n185 = flat-sequence {
                      tunnel: w259 -> [w263]
                      tunnel: w261 -> [w262]
                      tunnel: [w264] -> w260
                      tunnel: w260 -> [w269]
                      tunnel: w259 -> [w268]
                      frame #0 {
                        n186 = local read "ERROR"() -> (w265:errorcluster)
                        n187 = call "HVG_Write_DAC.vi"("Error_In"=w265, "DACnew"=w262, "ID"=w263) -> ("Error_Out"=w264:errorcluster)  [unwired: 2 in]
                      }
                      frame #1 {
                        n188 = call "HVG_Read_DAC.vi"("Error_In"=w269, "ID"=w268) -> ("Error_Out"=w266:errorcluster, "DACold"=w267:u16[])  [unwired: 2 in]
                        n189 = local write "DACOLD"(w267) -> ()
                        n190 = local write "ERROR"(w266) -> ()
                      }
                    }
                  }
                }
                n191 = local write "String"("SETTING DAC" ("String")) -> ()
              }
              frame #2 {
                n192 = local write "String"("AVERAGE..." ("String")) -> ()
                n193 = local read "ERROR"() -> (w271:errorcluster)
                n194 = call "HVG_avg_set.vi"("Error_In"=w271, "average"="AVG", "ID"=w272) -> ("Error_Out"=w270:errorcluster)  [unwired: 2 in]
                n195 = local write "ERROR"(w270) -> ()
              }
              frame #3 {
                n196 = local read "V_data"() -> (w289:cluster{dbl[], dbl[]}[])
                n197 = local read "I_data"() -> (w288:cluster{dbl[], dbl[]}[])
                n198 = local read "ERROR"() -> (w283:errorcluster)
                n199 = call "HVG_TPDOx_read.vi"("ID"=w282, "V_data_in"=w289, "I_data_in"=w288, "Error in"=w283) -> ("Data_read"=w285:bool, "V_data_out"=w287:cluster{dbl[], dbl[]}[], "I_data_out"=w286:cluster{dbl[], dbl[]}[], "Error out"=w284:errorcluster)  [unwired: 1 in]
                n200 = local write "TPD_read"(w285) -> ()
                n201 = local write "String"("HVMON" ("String")) -> ()
                n202 = local write "I_data"(w286) -> ()
                n203 = local write "V_data"(w287) -> ()
                n204 = local write "ERROR"(w284) -> ()
                n205 = call "HVG_GetDDisplay.vi"("I_data_out"=w287) -> ("Array"=w278:dbl[])
                n206 = call "HVG_GetDDisplay.vi"("I_data_out"=w286) -> ("Array"=w279:dbl[])
                n207 = local write "Currents"(w279) -> ()
                n208 = Multiply(x=w279, y=dbl[] [1000.0, 1000.0, 1000.0, 1000.0, 1000.0, 1000.0, 1000.0]) -> (x*y=w275:dbl[])
                "Currents 2" <- w275
                n209 = local write "Voltages"(w278) -> ()
                n210 = Wait (ms)(milliseconds to wait=u32 10) -> ()  [unwired: 1 out]
                n211 = Multiply(x=w278, y=dbl[] [1.0, 1.0, 1.0, 1.0, 1.0, 1.0, 1.0]) -> (x*y=w277:dbl[])
              }
              frame #4 {
                # "seconds at 1-1-2018"
                n212 = local read "refnum"() -> (w292:refnum<file>)
                n213 = local read "Write data"() -> (w299:bool)
                n214 = Get Date/Time In Seconds() -> (seconds since 1Jan1904=w297:timestamp)
                n215 = To Unsigned Long Integer(number=w297) -> (unsigned 32bit integer=w296:u32)
                n216 = Subtract(x=w296, y=u32 3597613200) -> (x-y=w295:u32)
                "time" <- w295
                n217 = Build Array (concatenate)(w295, w294, w293) -> (w298:dbl[])
                n218 = case shown="True" w299 {
                  tunnel: w298 -> [_ w303]
                  tunnel: w292 -> [_ w304]
                  frame False {
                  }
                  frame True {
                    n219 = local write "String"("WRITING FILE" ("String")) -> ()
                    n220 = call "Write_Open_File_int.vi"("delimiter (Tab)"=" ", "format (%.3f)"="%8d", "1D data"=w303, "refnum"=w304) -> ()  [unwired: 4 in, 1 out]
                    n221 = Wait (ms)(milliseconds to wait=u32 10 ("ms to write")) -> ()  [unwired: 1 out]
                  }
                }
              }
              frame #5 {
                n222 = local write "Write data"(FALSE) -> ()
              }
            }
            n223 = local read "ID"() -> (w246:u8)
          }
          frame #5 {
            n224 = local read "OvflThres"() -> (w307:u16)
            n225 = local read "DT"() -> (w309:u16)
            n226 = local read "dt"() -> (w308:u16)
            n227 = call "Trip_ParmsCheck.vi"("threshold"="CurrThres", "OvflThres"=w307, "dt"=w308, "DT"=w309) -> ("error"=w311:bool, "msg_out"=→"TripCtrl_msg":string)
            n228 = case shown="False" w311 {
              tunnel: w307 -> [w317 _]
              tunnel: "CurrThres" -> [w316 _]
              tunnel: w309 -> [w315 _]
              tunnel: w308 -> [w314 _]
              frame False {
                n229 = while {
                  tunnel: w317 -> [w359]
                  shift-right: [w357] -> _
                  shift-left: _ -> [w356]
                  stop <- TRUE stop-if-true
                  n230 = Equal?(x=w356, y=w359) -> (x = y?=w358:bool)
                  n231 = case shown="True" w358 {
                    tunnel: w359 -> [w361 _]
                    tunnel: [w361 w367] -> w357
                    tunnel: w356 -> [_ w367]
                    frame False {
                      n232 = local read "ERROR"() -> (w366:errorcluster)
                      n233 = local read "ID"() -> (w364:u8)
                      n234 = call "CO_SDO_write_1byte.vi"("ID"=w364, "Index"=u16 8232 ("CmdSpecifier"), "SubIndex"=u8 2, "error in"=w366, "Value"=w361) -> ("error out"=w365:errorcluster)  [unwired: 1 out]
                      n235 = local write "ERROR"(w365) -> ()
                    }
                    frame True {
                    }
                  }
                }
                n236 = while {
                  tunnel: w316 -> [w345]
                  shift-right: [w343] -> _
                  shift-left: _ -> [w342]
                  stop <- TRUE stop-if-true
                  n237 = Equal?(x=w342, y=w345) -> (x = y?=w344:bool)
                  n238 = case shown="True" w344 {
                    tunnel: w345 -> [w349 _]
                    tunnel: [w349 w355] -> w343
                    tunnel: w342 -> [_ w355]
                    frame False {
                      n239 = local read "ERROR"() -> (w354:errorcluster)
                      n240 = Multiply(x=100.0, y=w349) -> (x*y=w348:dbl)
                      n241 = local read "ID"() -> (w352:u8)
                      n242 = call "CO_SDO_write_2byte.vi"("Value"=w348, "error in (no error)"=w354, "SubIndex"=u8 1, "Index"=u16 8232 ("CmdSpecifier"), "ID"=w352) -> ("error out"=w353:errorcluster)  [unwired: 3 in, 1 out]
                      n243 = local write "ERROR"(w353) -> ()
                    }
                    frame True {
                    }
                  }
                }
                n244 = while {
                  tunnel: w315 -> [w333]
                  shift-right: [w331] -> _
                  shift-left: _ -> [w330]
                  stop <- TRUE stop-if-true
                  n245 = Equal?(x=w330, y=w333) -> (x = y?=w332:bool)
                  n246 = case shown="True" w332 {
                    tunnel: w333 -> [w335 _]
                    tunnel: [w335 w341] -> w331
                    tunnel: w330 -> [_ w341]
                    frame False {
                      n247 = local read "ERROR"() -> (w340:errorcluster)
                      n248 = local read "ID"() -> (w338:u8)
                      n249 = call "CO_SDO_write_2byte.vi"("Value"=w335, "error in (no error)"=w340, "SubIndex"=u8 3, "Index"=u16 8232 ("CmdSpecifier"), "ID"=w338) -> ("error out"=w339:errorcluster)  [unwired: 3 in, 1 out]
                      n250 = local write "ERROR"(w339) -> ()
                    }
                    frame True {
                    }
                  }
                }
                n251 = while {
                  tunnel: w314 -> [w321]
                  shift-right: [w319] -> _
                  shift-left: _ -> [w318]
                  stop <- TRUE stop-if-true
                  n252 = Equal?(x=w318, y=w321) -> (x = y?=w320:bool)
                  n253 = case shown="True" w320 {
                    tunnel: w321 -> [w323 _]
                    tunnel: [w323 w329] -> w319
                    tunnel: w318 -> [_ w329]
                    frame False {
                      n254 = local read "ERROR"() -> (w328:errorcluster)
                      n255 = local read "ID"() -> (w326:u8)
                      n256 = call "CO_SDO_write_2byte.vi"("Value"=w323, "error in (no error)"=w328, "SubIndex"=u8 4, "Index"=u16 8232 ("CmdSpecifier"), "ID"=w326) -> ("error out"=w327:errorcluster)  [unwired: 3 in, 1 out]
                      n257 = local write "ERROR"(w327) -> ()
                    }
                    frame True {
                    }
                  }
                }
                n258 = local write "String"("CHECKING TRIPS" ("String")) -> ()
              }
              frame True {
              }
            }
          }
          frame #6 {
            n259 = flat-sequence {
              tunnel: [w394] -> w368
              tunnel: w368 -> [w399]
              frame #0 {
                n260 = while {
                  shift-right: [w372] -> _
                  shift-left: _ -> [w371]
                  tunnel: "Trip Control" -> [w370]
                  stop <- TRUE stop-if-true
                  n261 = Equal?(x=w371, y=w370) -> (x = y?=w373:bool)
                  n262 = case shown="False" w373 {
                    tunnel: w370 -> [w380 _]
                    tunnel: [w380 w383] -> w372
                    tunnel: w371 -> [_ w383]
                    frame False {
                      w375 = u8 5 ("SubIndex")
                      w378 = u16 8232 ("CmdSpecifier")
                      n263 = local read "ERROR"() -> (w382:errorcluster)
                      n264 = Boolean To (0,1)(Boolean=w380) -> (0, 1=w381:i16)
                      n265 = local read "ID"() -> (w379:u8)
                      n266 = call "CO_SDO_write_1byte.vi"("ID"=w379, "Index"=w378, "SubIndex"=w375, "error in"=w382, "Value"=w381) -> ("error out"=w376:errorcluster)  [unwired: 1 out]
                      n267 = call "CO_SDO_read_xbyte.vi"("error in"=w376, "SubIndex"=w375, "Index"=w378, "ID"=w379) -> ("error out"=w377:errorcluster)  [unwired: 2 in, 3 out]
                      n268 = local write "ERROR"(w377) -> ()
                    }
                    frame True {
                    }
                  }
                }
              }
              frame #1 {
                n269 = case shown="True" "SpsAcc" {
                  tunnel: [u16 40 ("DT") u16 1000 ("DT")] -> w387
                  tunnel: [u16 4 ("dt") u16 20 ("dt")] -> w386
                  tunnel: [u8 10 ("OvflThres") u8 25 ("OvflThres")] -> w385
                  frame False {
                  }
                  frame True {
                  }
                }
                n270 = local write "OvflThres"(w385) -> ()
                n271 = local write "DT"(w387) -> ()
                n272 = local write "dt"(w386) -> ()
              }
              frame #2 {
                n273 = local read "ID"() -> (w396:u8)
                n274 = local read "ERROR"() -> (w398:errorcluster)
                n275 = call "TC_GetOvflCnt.vi"("ID"=w396, "Error_Status_in"=w398) -> ("ChOvfl"=→"OVC":u32[], "Trip Check status"=w394:u16, "Error_Status_out"=w397:errorcluster)
                "Trip Status" <- w394
                n276 = local write "ERROR"(w397) -> ()
              }
              frame #3 {
                n277 = case shown="0, Default" w399 {
                  frame 0, Default {
                  }
                  frame 3 {
                    n278 = local write "ON"(FALSE ("ON")) -> ()
                  }
                }
              }
            }
          }
          frame #7 {
            n279 = local read "ERROR"() -> (w424:errorcluster)
            n280 = local read "ID"() -> (w425:u8)
            n281 = call "CO_NodeGuard.vi"("error in (no error)"=w424, "ID"=w425) -> ("error out"=w423:errorcluster, "Operational"=w419:bool, "PreOperational"=w420:bool)  [unwired: 3 in, 2 out]
            n282 = local read "ID"() -> (w426:u8)
            n283 = call "HVG_Poll_Regs.vi"("Error in"=w423, "ID"=w426) -> ("Error out"=w422:errorcluster, "HVG module status"=w414:T3)  [unwired: 1 in]
            n284 = local write "PreOperational"(w420) -> ()
            n285 = local write "Operational"(w419) -> ()
            n286 = local write "ERROR"(w422) -> ()
            n287 = Unbundle By Name(w414) -> ("Safety switch"=w413:bool, "HV disable switch"=w412:bool, "HV_on"=w402:bool[], "I_gain_x10"=→"I_gain_x10":bool[], "FSM_status"=→"FSM_status":u16, "0x2020"=→"Power Supply Levels":dbl[], "Tstep"=→"Tstep [ms]":u16, "Tramp"=→"Tramp [s]":u16, "Average"=→"avg":i16, "Current AGC"=→"Current_AGC_led":bool, "Wiper"=→"Wiper":i16[], "Slope [V/s]"=→"slope read":i16)
            "HV_on" <- w402
            n288 = Not(x=w413) -> (.not. x?=→"Safety switch":bool)
            n289 = Not(x=w412) -> (.not. x?=w417:bool)
            "HV enable switch" <- w417
            n290 = Or Array Elements(Boolean array=w402) -> (logical OR=→"HV_flag":bool)
            n291 = Not(x=w417) -> (.not. x?=w416:bool)
            n292 = And(x="HV enable switch old", y=w416) -> (x .and. y?=w418:bool)
            n293 = case shown="True" w418 {
              frame False {
              }
              frame True {
                n294 = local write "ON"(FALSE) -> ()
              }
            }
          }
          frame #8 {
            n295 = local read "Voltages"() -> (w428:dbl[])
            n296 = Index Array(array=w428, index=6) -> (element=w437:dbl)
            "Vd" <- w437
            n297 = Index Array(array=w428, index=5) -> (element=w433:dbl)
            "G1" <- w433
            n298 = Index Array(array=w428, index=4) -> (element=w436:dbl)
            "Vt1" <- w436
            n299 = Index Array(array=w428, index=3) -> (element=w432:dbl)
            "G2" <- w432
            n300 = Index Array(array=w428, index=2) -> (element=w435:dbl)
            "Vt2" <- w435
            n301 = Index Array(array=w428, index=1) -> (element=w431:dbl)
            "G3" <- w431
            n302 = Index Array(array=w428, index=0) -> (element=w434:dbl)
            "Vi" <- w434
            n303 = Build Array(w433, w432, w431) -> (w438:dbl[])
            n304 = Add Array Elements(numeric array=w438) -> (sum=→"Gain":dbl)
            n305 = local read "gt2"() -> (w451:dbl)
            n306 = local read "gd"() -> (w449:dbl)
            n307 = Divide(x=w435, y=w451) -> (x/y=w454:dbl)
            "Et2" <- w454
            n308 = Divide(x=w437, y=w449) -> (x/y=w441:dbl)
            "Ed" <- w441
            n309 = local read "gt1"() -> (w452:dbl)
            n310 = local read "gi"() -> (w450:dbl)
            n311 = Divide(x=w434, y=w450) -> (x/y=w455:dbl)
            "Ei" <- w455
            n312 = Divide(x=w436, y=w452) -> (x/y=w453:dbl)
            "Et1" <- w453
            n313 = global write "variables.vi" "ED"(w441) -> ()
            n314 = global write "variables.vi" "ET1"(w453) -> ()
            n315 = global write "variables.vi" "ET2"(w454) -> ()
            n316 = global write "variables.vi" "EI"(w455) -> ()
            n317 = Bundle(w441, w453, w454, w455) -> (→"Fields kV/cm":cluster{dbl, dbl, dbl, dbl})  [unwired: 1 in]
            n318 = Bundle(w433, w432, w431) -> (→"GEM Volt":cluster{dbl, dbl, dbl})  [unwired: 1 in]
            n319 = local write "String"("FILLING  HISTOS" ("String")) -> ()
          }
          frame #9 {
            n320 = local read "Currents"() -> (w465:dbl[])
            n321 = Index Array(array=w465, index=6) -> (element=w463:dbl)
            n322 = Index Array(array=w465, index=5) -> (element=w462:dbl)
            n323 = Index Array(array=w465, index=4) -> (element=w461:dbl)
            n324 = Index Array(array=w465, index=3) -> (element=w460:dbl)
            n325 = Index Array(array=w465, index=2) -> (element=w459:dbl)
            n326 = Index Array(array=w465, index=1) -> (element=w458:dbl)
            n327 = Index Array(array=w465, index=0) -> (element=w457:dbl)
            n328 = Bundle(w463, w462, w461, w460, w459, w458, w457) -> (→"Currents micro":cluster{dbl, dbl, dbl, dbl, dbl, dbl, dbl})  [unwired: 1 in]
            n329 = local write "String"("FILLING  HISTOS" ("String")) -> ()
          }
        }
      }
    }
    frame #3 {
      n330 = flat-sequence {
        frame #0 {
          n331 = global read "GlobalData.vi" "CAN Handle"() -> (w474:i32)
          n332 = call "kvCanBusOff.vi"("Channel Handle (input only)"=w474) -> ("error out"=w473:errorcluster, "Channel Handle (ouput only)"=w475:i32)  [unwired: 1 in]
          n333 = call "kvCanClose.vi"("error in (no error)"=w473, "Channel Handle (input only)"=w475) -> ("error out"=w476:errorcluster)
          n334 = local write "ERROR"(w476) -> ()
        }
        frame #1 {
          w479 = u16 1 items=["no dialog", "OK message", "continue or stop message"] ("type of dialog (OK msg:1)")
          w478 = string[] ["Cannot open CAN channel", "Invalid handle"]  # [user-defined descriptions]
          w477 = i32[] [-3, -10]  # [user-defined codes]
          n335 = call <vilib>:"General Error Handler.vi"("[user-defined codes]"=w477, "[user-defined descriptions]"=w478, "type of dialog (OK msg:1)"=w479) -> ()  [unwired: 8 in, 5 out]
        }
        frame #2 {
          n336 = local read "refnum"() -> (w480:refnum<file>)
          n337 = Close File(refnum=w480) -> ()  [unwired: 1 in, 2 out]
        }
      }
    }
  }
